vi "Cycle.vi"(8 "error in (no error)":errorcluster, 11 "BehaviorClassification In":refnum<class "ClassDiscrimination.lvclass">) -> (0 "error out":errorcluster, 3 "BehaviorClassification Out":refnum<class "ClassDiscrimination.lvclass">)   [LabVIEW 2011, in "ClassDiscrimination.lvclass"]
uses:
  ClassDiscrimination.lvclass
  MatlabExperiment/MatlabExperiment.lvclass
panel:
  in  "Eye Params":dbl[](array[numeric])
  out "XY Graph":cluster{dbl[], dbl[]}(graph)
  in  "RewardAmount":dbl=50.0
  in  "FixationRadius":dbl=50.0
  out "Timeouts":T1={"Intertrial"=1000.0, "AcquireFixation"=1000.0, "HoldFixation"=300.0, "DelayPeriod"=1000.0, "ResponsePeriod"=1000.0}
  out "ExperimentStats":T2
  out "Cycles":dbl
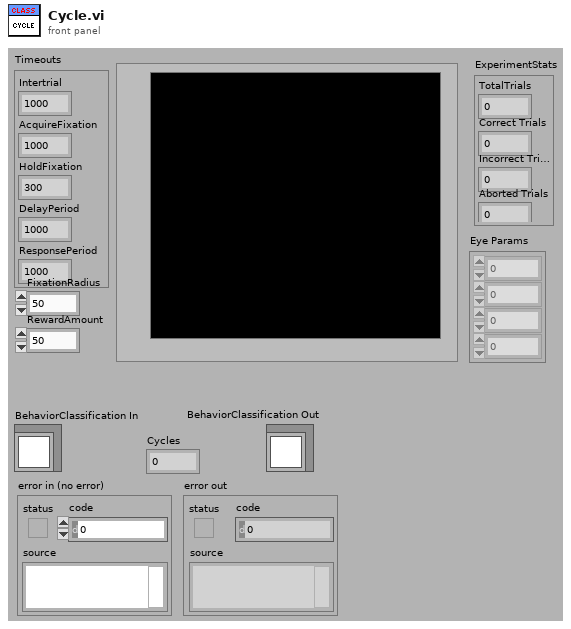
[diagram p1: front panel]
types:
  T1 = cluster{"Intertrial":dbl, "AcquireFixation":dbl, "HoldFixation":dbl, "DelayPeriod":dbl, "ResponsePeriod":dbl}
  T2 = cluster{"TotalTrials":dbl, "Correct Trials":dbl, "Incorrect Trials":dbl, "Aborted Trials":dbl}
  T3 = cluster{"TotalTrials":u32, "Correct Trials":u32, "Incorrect Trials":u32, "Aborted Trials":u32}
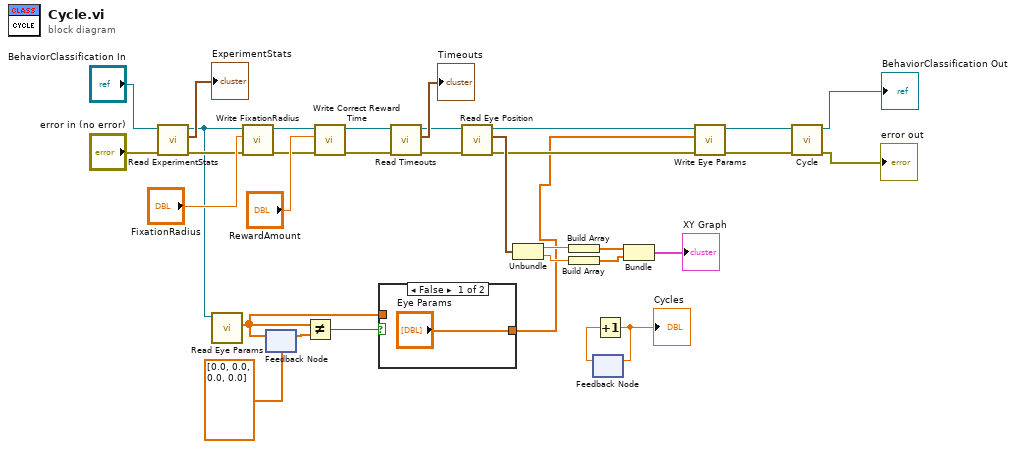
[diagram p0: block diagram]
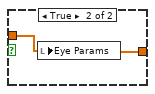
[diagram p2: hidden frame]
diagram:
  n1 = call-dynamic "Read ExperimentStats.vi"("error in (no error)"="error in (no error)", "TrialBasedExperiment in"="BehaviorClassification In") -> ("error out"=w23:errorcluster, "ExperimentStats"=→"ExperimentStats":T3, "TrialBasedExperiment out"=w6:refnum<class "ClassDiscrimination.lvclass">)  [unwired: 7 in]
  n2 = call-dynamic "Read Eye Params.vi"("TrialBasedExperiment in"=w6) -> ("Eye Params"=w3:dbl[])  [unwired: 8 in, 2 out]
  n3 = call-dynamic "Write FixationRadius.vi"("error in (no error)"=w23, "FixationRadius"="FixationRadius", "MatlabExperiment in"=w6) -> ("error out"=w22:errorcluster, "MatlabExperiment out"=w25:refnum<class "ClassDiscrimination.lvclass">)  [unwired: 7 in]
  n4 = feedback-in #1(w3) -> ()
  n5 = feedback #1(dbl[] [0.0, 0.0, 0.0, 0.0] ("Eye Params")) -> (w5:dbl[])
  n6 = Not Equal?(x=w3, y=w5) -> (x != y?=w4:bool)
  n7 = call-dynamic "Write Correct Reward Time.vi"("error in (no error)"=w22, "Correct Reward Time"="RewardAmount", "MatlabExperiment in"=w25) -> ("error out"=w21:errorcluster, "MatlabExperiment out"=w24:refnum<class "ClassDiscrimination.lvclass">)  [unwired: 7 in]
  n8 = case shown="False" w4 {
    tunnel: w3 -> [_ w35]
    tunnel: ["Eye Params" w35] -> w2
    frame False {
    }
    frame True {
      n9 = local write "Eye Params"(w35) -> ()
    }
  }
  n10 = call-dynamic "Read Timeouts.vi"("error in (no error)"=w21, "TrialBasedExperiment in"=w24) -> ("error out"=w13:errorcluster, "Timeouts"=→"Timeouts":T1, "TrialBasedExperiment out"=w14:refnum<class "ClassDiscrimination.lvclass">)  [unwired: 7 in]
  n11 = call-dynamic "Read Eye Position.vi"("error in (no error)"=w13, "TrialBasedExperiment in"=w14) -> ("error out"=w11:errorcluster, "Eye Position"=w20:cluster{"Horizontal":dbl, "Vertical":dbl}, "TrialBasedExperiment out"=w12:refnum<class "ClassDiscrimination.lvclass">)  [unwired: 7 in]
  n12 = Unbundle(w20) -> ("Horizontal"=w19:dbl, "Vertical"=w18:dbl)
  n13 = Build Array(w19) -> (w17:dbl[])
  n14 = Build Array(w18) -> (w16:dbl[])
  n15 = feedback #2() -> (w32:dbl)  [unwired: 1 in]
  n16 = Increment(x=w32) -> (x+1=w33:dbl)
  "Cycles" <- w33
  n17 = feedback-in #2(w33) -> ()
  n18 = Bundle(w17, w16) -> (→"XY Graph":cluster{dbl[], dbl[]})  [unwired: 1 in]
  n19 = call-dynamic "Write Eye Params.vi"("error in (no error)"=w11, "Eye Params"=w2, "TrialBasedExperiment in"=w12) -> ("error out"=w9:errorcluster, "TrialBasedExperiment out"=w10:refnum<class "ClassDiscrimination.lvclass">)  [unwired: 7 in]
  n20 = call-parent "Cycle.vi"("error in (no error)"=w9, "MatlabExperiment In"=w10) -> ("error out"=→"error out":errorcluster, "MatlabExperiment Out"=→"BehaviorClassification Out":refnum<class "ClassDiscrimination.lvclass">)  [unwired: 8 in]
